vi "PreProcess.vi"(8 "error in (no error)":errorcluster, 10 "Variant in":variant, 11 "ONNX YOLO Class in":refnum<class "ONNX YOLO Class.lvclass">) -> (0 "error out":errorcluster, 2 "Variant out":variant, 3 "ONNX YOLO Class out":refnum<class "ONNX YOLO Class.lvclass">)   [LabVIEW 2017, in "ONNX YOLO Class Library.lvlib" / "ONNX YOLO Class.lvclass"]
uses:
  ONNX YOLO Class.lvclass
  ONNX YOLO Class.lvclass/ONNX YOLO Class.ctl
  <vilib>/picture/picture.llb/imagedata.ctl
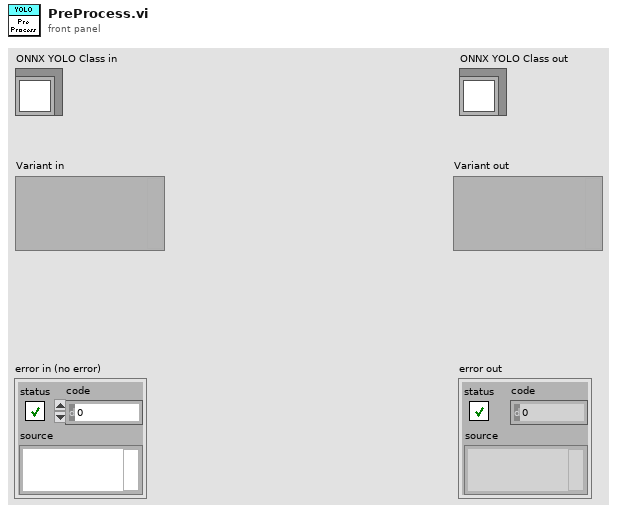
[diagram p1: front panel]
types:
  T1 = typedef "imagedata.ctl" = cluster{"image type":i32, "image depth":i32, "image":u8[], "mask":u8[], "colors":u32[], "Rectangle":cluster{"left":i16, "top":i16, "right":i16, "bottom":i16}}
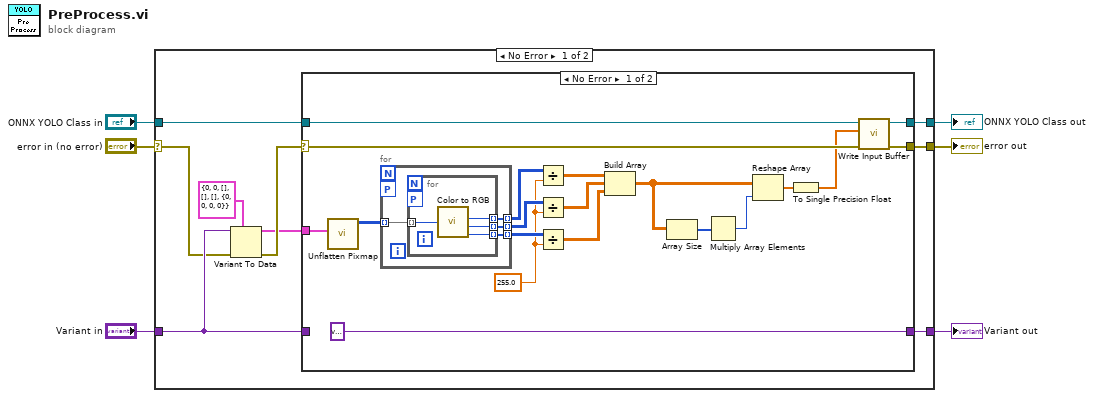
[diagram p0: block diagram]
diagram:
  n1 = case shown="No Error" "error in (no error)" {
    selector: "error in (no error)" -> [w7 w47]
    tunnel: "ONNX YOLO Class in" -> [w12 w48]
    tunnel: [w11 w48] -> w5
    tunnel: [w10 w47] -> w4
    tunnel: "Variant in" -> [w9 w46]
    tunnel: [w8 w46] -> w2
    frame No Error {
      n2 = Variant To Data(error in=w7, type=T1 {"image type"=0, "image depth"=0, "image"=[], "mask"=[], "colors"=[], "Rectangle"={"left"=0, "top"=0, "right"=0, "bottom"=0}} ("image data"), Variant=w9) -> (data=w13:T1, error out=w14:errorcluster)
      n3 = case shown="No Error" w14 {
        selector: w14 -> [w19 w44]
        tunnel: w13 -> [w22 _]
        tunnel: w12 -> [w21 w45]
        tunnel: [w20 w45] -> w11
        tunnel: [w18 w44] -> w10
        tunnel: w9 -> [_ w43]
        tunnel: [variant w43] -> w8
        frame No Error {
          w23 = 255.0 ("y")
          n4 = call <vilib>:"Unflatten Pixmap.vi"("image data"=w22) -> ("24-bit pixmap"=w34:u32[][])  [unwired: 10 out]
          n5 = for {
            tunnel: w34 -> [w38] mode=indexing
            tunnel: [w37] -> w24 mode=indexing
            tunnel: [w36] -> w25 mode=indexing
            tunnel: [w35] -> w26 mode=indexing
            workers-P: _ -> [_]
            n6 = for {
              tunnel: w38 -> [w39] mode=indexing
              tunnel: [w42] -> w37 mode=indexing
              tunnel: [w41] -> w36 mode=indexing
              tunnel: [w40] -> w35 mode=indexing
              workers-P: _ -> [_]
              n7 = call <vilib>:"Color to RGB.vi"("Color"=w39) -> ("R"=w42:u8, "G"=w41:u8, "B"=w40:u8)  [unwired: 1 out]
            }
          }
          n8 = Divide(x=w24, y=w23) -> (x/y=w27:dbl[][])
          n9 = Divide(x=w25, y=w23) -> (x/y=w28:dbl[][])
          n10 = Divide(x=w26, y=w23) -> (x/y=w29:dbl[][])
          n11 = Build Array(w27, w28, w29) -> (w31:dbl[][][])
          n12 = Array Size(array=w31) -> (size(s)=w30:i32[])
          n13 = Multiply Array Elements(1:w30) -> (0:w32:i32)
          n14 = Reshape Array(w31, w32) -> (w33:dbl[])
          n15 = To Single Precision Float(number=w33) -> (single precision float=w16:sgl[])
          n16 = call-dynamic "Write Input Buffer.vi"("error in (no error)"=w19, "Input Buffer"=w16, "ONNX Class in"=w21) -> ("error out"=w18:errorcluster, "ONNX Class out"=w20:refnum<class "ONNX YOLO Class.lvclass">)  [unwired: 7 in]
        }
        frame Error {
        }
      }
    }
    frame Error {
    }
  }
  "error out" <- w4
  "ONNX YOLO Class out" <- w5
  "Variant out" <- w2
